vi "Current - SW-Timed Input.vi"() -> ()   [LabVIEW 2022 SP3]
doc: "This example demonstrates how to continuously acquire current measurements using software-timing with a DAQmx device.\n\nFor instructions on how to connect your signals to the DAQ device, refer to your device documentation."
uses:
  <vilib>/Utility/error.llb/DialogType.ctl
  <vilib>/DAQmx/read.llb/DAQmx Read (Analog 1D Wfm NChan 1Samp).vi
  <vilib>/DAQmx/create/channels.llb/DAQmx Create Channel (AI-Current-Basic).vi
  <vilib>/DAQmx/miscellaneous.llb/DAQmx Fill In Error Info.vi
panel:
  in  "Loop Time (ms)":u32=100
  in  "Shunt Value (Ohms)":dbl=249.0 format="%0.2f"
  in  "Shunt Resistor":i32(ring)=-1 items=["default"=-1, "Internal"=10200, "External"=10167]
  in  "Stop":bool
  out "Waveform Chart":waveform(dbl)[](graph)
  in  "Max Current":dbl=0.02
  in  "Min Current":dbl
  in  "Physical Channel":tag="Dev1/ai0"
  # "Channel Settings"
  # "Acquired Data"
  # "Timing Settings"
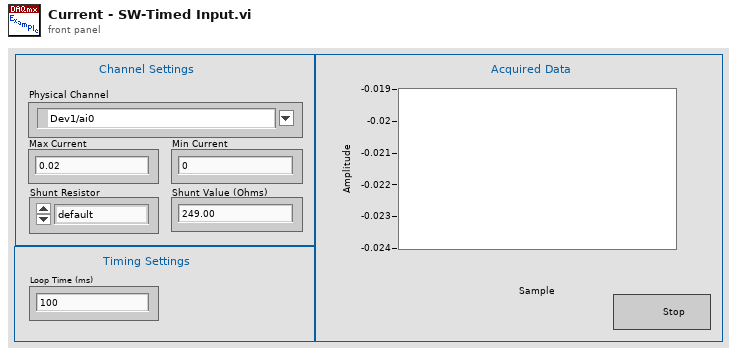
[diagram p1: front panel]
types:
  T1 = typedef "DialogType.ctl" = u16
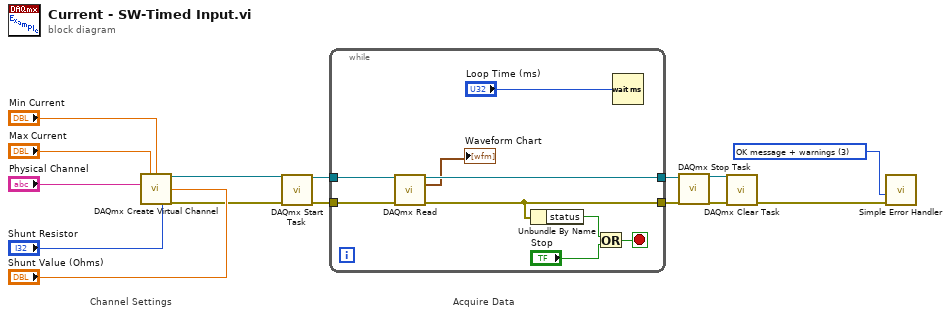
[diagram p0: block diagram]
diagram:
  w1 = T1 3 items=["no dialog", "OK message", "continue or stop message", "OK message + warnings", "continue/stop + warnings"] ("type of dialog (OK msg:1)")
  # "Acquire Data"
  # "Channel Settings"
  n1 = call-poly <vilib>:"DAQmx Create Virtual Channel.vi"("maximum value"="Max Current", "minimum value"="Min Current", "physical channels"="Physical Channel", "external shunt resistor value"="Shunt Value (Ohms)", "shunt resistor location"="Shunt Resistor") -> ("task out"=w7:refnum<k21>, "error out"=w6:errorcluster)  [unwired: 9 in]
  n2 = call <vilib>:"DAQmx Start Task.vi"("task/channels in"=w7, "error in"=w6) -> ("task out"=w15:refnum<k21>, "error out"=w14:errorcluster)  [unwired: 12 in]
  n3 = while {
    tunnel: w15 -> [w24]
    tunnel: w14 -> [w23]
    tunnel: [w20] -> w4
    tunnel: [w21] -> w5
    stop <- w22 stop-if-true
    n4 = call-poly <vilib>:"DAQmx Read.vi"("task/channels in"=w24, "error in"=w23) -> ("task out"=w21:refnum<k21>, "data"=→"Waveform Chart":waveform(dbl)[], "error out"=w20:errorcluster)  [unwired: 11 in]
    n5 = Unbundle By Name(w20) -> ("status"=w19:bool)
    n6 = Or(x=w19, y="Stop") -> (x .or. y?=w22:bool)
    n7 = Wait (ms)(milliseconds to wait="Loop Time (ms)") -> ()  [unwired: 1 out]
  }
  n8 = call <vilib>:"DAQmx Stop Task.vi"("task/channels in"=w5, "error in"=w4) -> ("task out"=w3:refnum<k21>, "error out"=w2:errorcluster)  [unwired: 12 in]
  n9 = call <vilib>:"DAQmx Clear Task.vi"("task in"=w3, "error in"=w2) -> ("error out"=w13:errorcluster)  [unwired: 13 in]
  n10 = call <vilib>:"Simple Error Handler.vi"("type of dialog (OK msg:1)"=w1, "error in (no error)"=w13) -> ()  [unwired: 3 in, 5 out]
